vi "temp_overlay.vi"() -> ()   [LabVIEW 2018]
uses:
  <vilib>/userdefined/High Color/IMAQdx.ctl
  <vilib>/vision/driver/NI_Vision_Acquisition_Software.lvlib
  <vilib>/vision/NI_Vision_Development_Module.lvlib
panel:
  out "색 상자":u32(colorbox)
  in  "숫자형":u8
  out "Graphe d'intensité":dbl[][](graph)
  in  "Size(x)":i16=600
  in  "Size(y)":i16=1000
  in  "Position":cluster{"x-coord":i32, "y-coord":i32}={"x-coord"=100, "y-coord"=50}
  in  "Transparency Factor":sgl(slide)=0.5 scale=0.0..1.0
  in  "Camera":T1="cam1"
  in  "stop":bool
  out "Cam  2":T2(plugin-control)
  in  "stop 3":bool
  out "Temperature 2":dbl[][](graph)
  in  "2D 배열 2":dbl[][](array[numeric])=[[5.0, 0.0, 0.0, 0.0, 0.0, 0.0, 0.0, 0.0, 0.0, 0.0], [0.0, 0.0, 0.0, 0.0, 0.0, 0.0, 0.0, 0.0, 0.0, 0.0], [0.0, 0.0, 0.0, 0.0, 0.0, 0.0, 0.0, 0.0, 0.0, 0.0], [0.0, 10.0, 0.0, 0.0, 0.0, 0.0, 0.0, 0.0, 0.0, 0.0], [0.0, 0.0, 0.0, 0.0, 0.0, 0.0, 0.0, 0.0, 0.0, 0.0], [0.0, 0.0, 0.0, 20.0, 0.0, 0.0, 0.0, 0.0, 0.0, 0.0], [0.0, 0.0, 0.0, 0.0, 0.0, 0.0, 0.0, 40.0, 0.0, 0.0], [0.0, 0.0, 0.0, 0.0, 0.0, 0.0, 0.0, 0.0, 0.0, 0.0], [0.0, 0.0, 0.0, 0.0, 30.0, 0.0, 0.0, 0.0, 0.0, 0.0], [0.0, 0.0, 0.0, 0.0, 0.0, 0.0, 0.0, 0.0, 0.0, 50.0]]
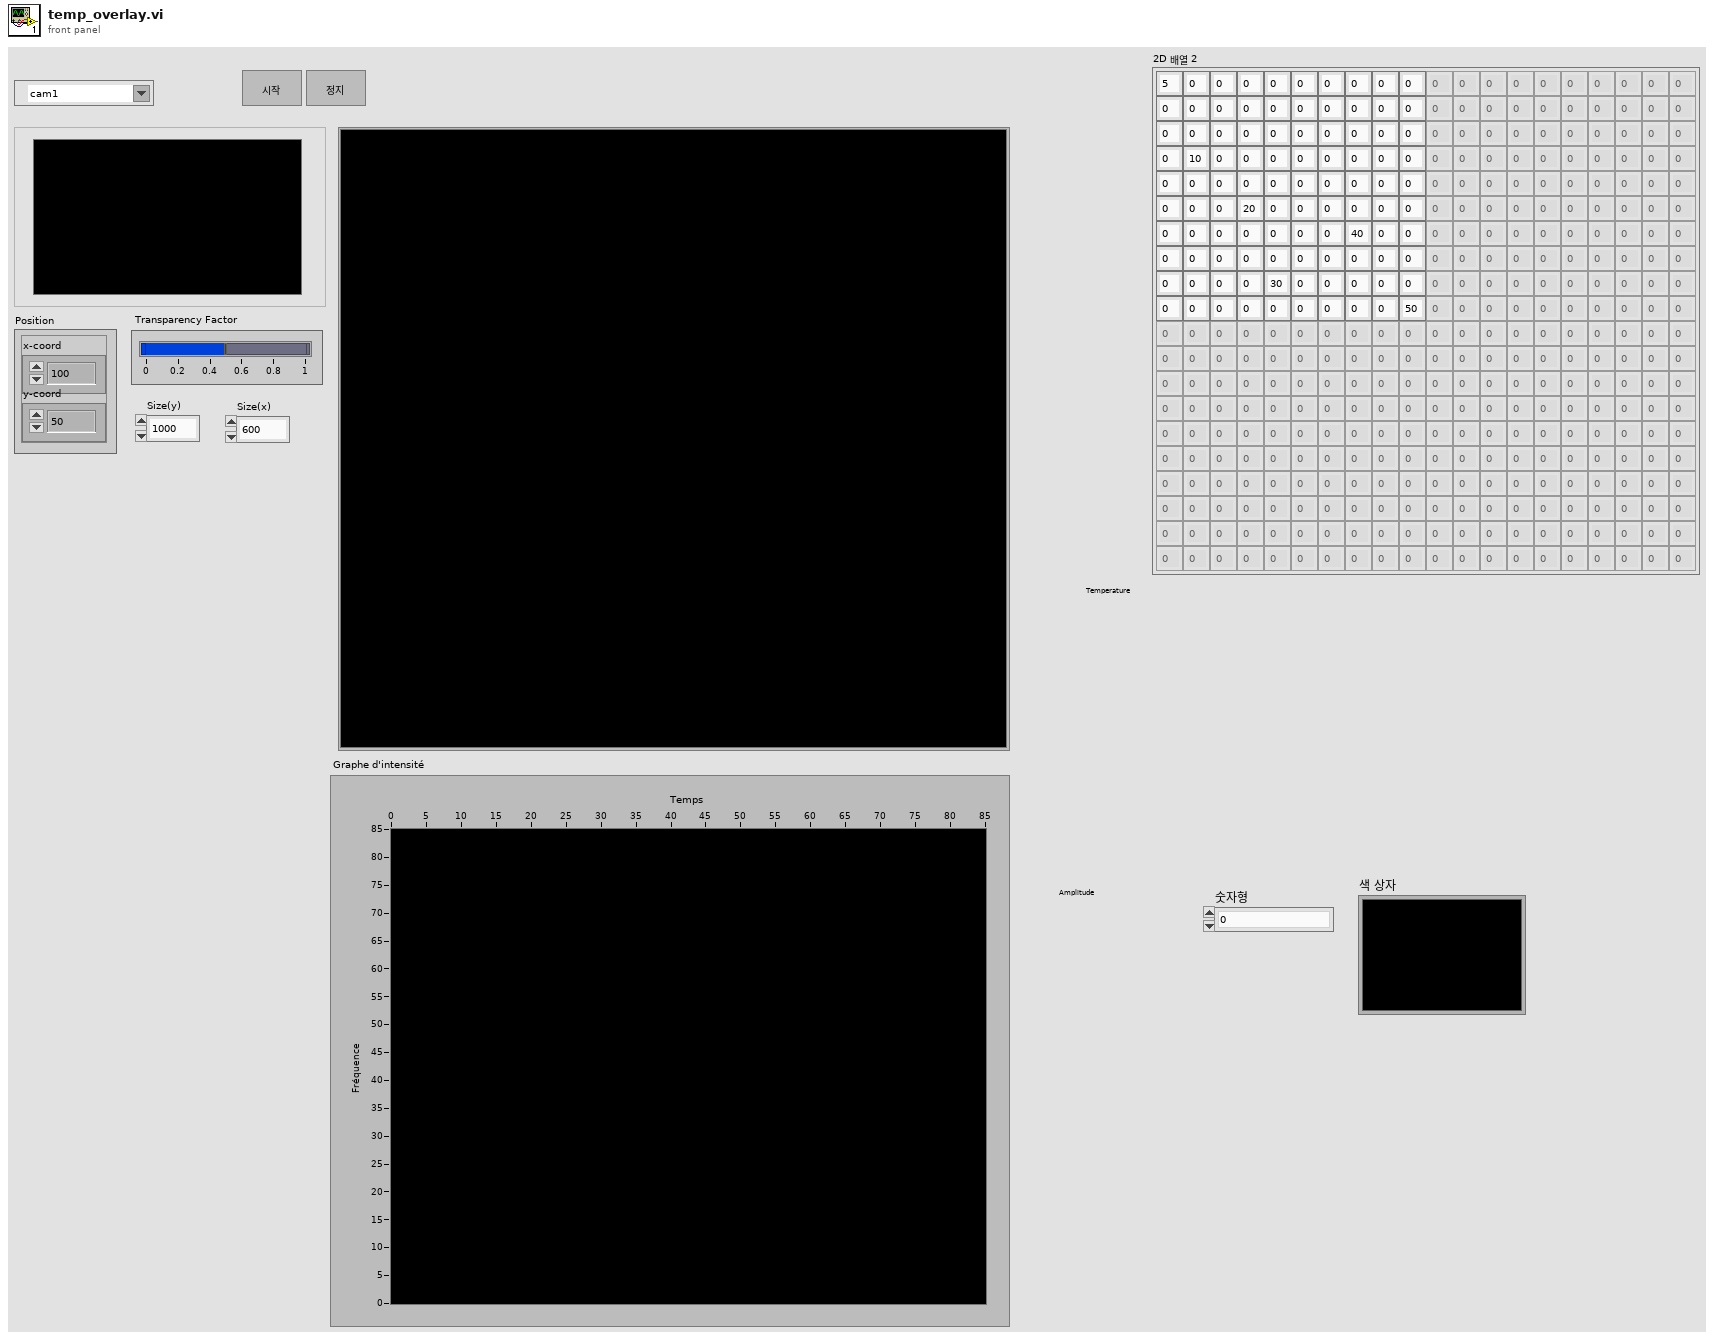
[diagram p1: front panel]
types:
  T1 = typedef "IMAQdx.ctl" = refnum<k21>
  T2 = typedef "IMAQ Image.ctl" = refnum<image>
  T3 = typedef "imagedata.ctl" = cluster{"image type":i32, "image depth":i32, "image":u8[], "mask":u8[], "colors":u32[], "Rectangle":cluster{"left":i16, "top":i16, "right":i16, "bottom":i16}}
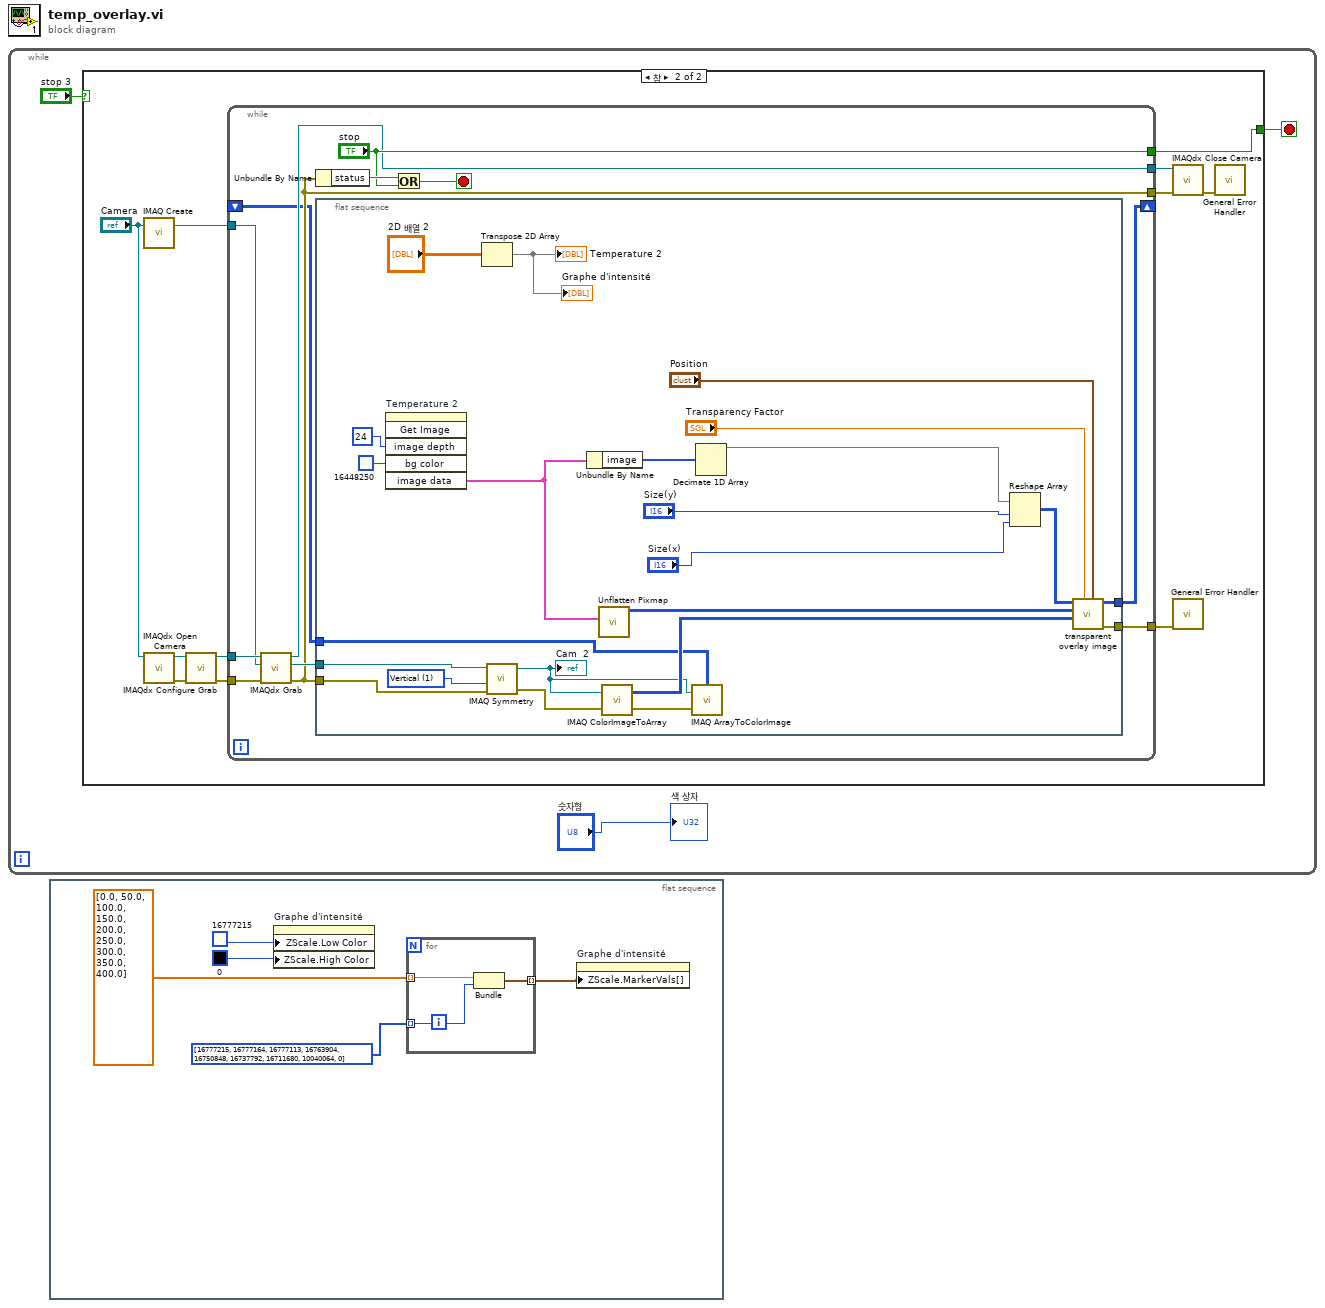
[diagram p0: block diagram]
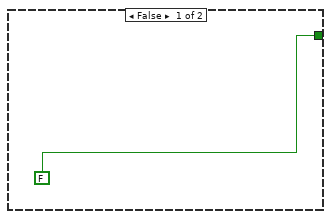
[diagram p2: hidden frame]
diagram:
  n1 = while {
    stop <- w2 stop-if-true
    n2 = case shown="참" "stop 3" {
      tunnel: [FALSE ("stop") w6] -> w2
      frame False {
      }
      frame True {
        n3 = call "IMAQ Create"("Image Name"="Camera") -> ("New Image"=w15:T2)  [unwired: 3 in, 2 out]
        n4 = call <vilib>:"IMAQdx Open Camera.vi"("Session In"="Camera") -> ("error out"=w9:errorcluster, "Session Out"=w11:T1)  [unwired: 2 in, 7 out]
        n5 = call <vilib>:"IMAQdx Configure Grab.vi"("error in"=w9, "Session In"=w11) -> ("error out"=w7:errorcluster, "Session Out"=w8:T1)  [unwired: 1 in, 7 out]
        n6 = while {
          tunnel: [w22] -> w14
          tunnel: w7 -> [w24]
          tunnel: w8 -> [w25]
          tunnel: [w19] -> w13
          tunnel: w15 -> [w21]
          tunnel: ["stop"] -> w6
          tunnel: [w16] -> w5
          shift-right: [w18] -> _
          shift-left: _ -> [w17]
          stop <- w27 stop-if-true
          n7 = call <vilib>:"IMAQdx Grab.vi"("error in"=w24, "Image In"=w21, "Session In"=w25) -> ("error out"=w19:errorcluster, "Image Out"=w20:T2, "Session Out"=w22:T1)  [unwired: 5 in, 1 out]
          n8 = Unbundle By Name(w19) -> ("status"=w26:bool)
          n9 = flat-sequence {
            tunnel: w20 -> [w49]
            tunnel: w19 -> [w40]
            tunnel: [w37] -> w18
            tunnel: w17 -> [w36]
            tunnel: [w34] -> w16
            frame #0 {
              w50 = u32 1 items=["Horizontal", "Vertical", "Central", "1st Diagonal", "2nd Diagonal"] ("Type of Symmetry")
              n10 = invoke on="Temperature 2" class="IntGraph (엄격한)" method="Get Image"("image depth"=24 ("이미지 농도"), "bg color"=u32 16448250 ("배경색")) -> ("image data"=w31:T3)  [unwired: 4 in, 5 out]
              n11 = Transpose 2D Array(2D array="2D 배열 2") -> (transposed array=→"Temperature 2" →"Graphe d'intensité":dbl[][])
              n12 = call "IMAQ Symmetry"("error in (no error)"=w40, "Type of Symmetry"=w50, "Image Src"=w49) -> ("error out"=w39:errorcluster, "Image Dst Out"=w45:T2)  [unwired: 2 in]
              "Cam  2" <- w45
              n13 = Unbundle By Name(w31) -> ("image"=w44:u8[])
              n14 = call <vilib>:"Unflatten Pixmap.vi"("image data"=w31) -> ("24-bit pixmap"=w41:u32[][])  [unwired: 4 in, 6 out]
              n15 = call "IMAQ ColorImageToArray"("Image"=w45, "error in (no error)"=w39) -> ("Image Pixels (U32)"=w46:u32[][], "error out"=w35:errorcluster)  [unwired: 2 in, 1 out]
              n16 = call "IMAQ ArrayToColorImage"("Image Pixels (U32)"=w36, "Image"=w45, "error in (no error)"=w35) -> ()  [unwired: 2 in, 2 out]
              n17 = Decimate 1D Array(w44) -> (w43:u8[])  [unwired: 3 out]
              n18 = Reshape Array(w43, "Size(y)", "Size(x)") -> (w42:u8[][])
              n19 = call "transparent overlay image.vi"("Coordinates of Overlay"="Position", "Transparency Factor"="Transparency Factor", "Image"=w46, "Overlay"=w41, "Alpha Values (Transparency)"=w42) -> ("error out"=w34:errorcluster, "Image Out"=w37:u32[][])  [unwired: 5 in]
            }
          }
          n20 = Or(x=w26, y="stop") -> (x .or. y?=w27:bool)
        }
        n21 = call <vilib>:"IMAQdx Close Camera.vi"("error in"=w13, "Session In"=w14) -> ("error out"=w12:errorcluster)  [unwired: 9 out]
        n22 = call <vilib>:"General Error Handler.vi"("error in (no error)"=w5) -> ()  [unwired: 2 in, 13 out]
        n23 = call <vilib>:"General Error Handler.vi"("error in (no error)"=w12) -> ()  [unwired: 2 in, 13 out]
      }
    }
    "색 상자" <- "숫자형"
  }
  n24 = flat-sequence {
    frame #0 {
      n25 = property on="Graphe d'intensité" class="IntGraph (엄격한)"("ZScale.Low Color"=u32 16777215 ("Boîte de couleur"), "ZScale.High Color"=u32 0 ("Boîte de couleur")) -> ()  [unwired: 2 in, 2 out]
      n26 = for {
        tunnel: u32[] [16777215, 16777164, 16777113, 16763904, 16750848, 16737792, 16711680, 10040064, 0] ("Couleurs  2") -> [w58] mode=indexing
        tunnel: [w57] -> w51 mode=indexing
        tunnel: dbl[] [0.0, 50.0, 100.0, 150.0, 200.0, 250.0, 300.0, 350.0, 400.0] -> [w56] mode=indexing
        n27 = Bundle(w56, "Boîte de couleur"=w58) -> (w57:cluster{dbl, "Boîte de couleur":u32})  [unwired: 1 in]
      }
      n28 = property on="Graphe d'intensité" class="IntGraph (엄격한)"("ZScale.MarkerVals[]"=w51) -> ()  [unwired: 2 in, 2 out]
    }
  }
